vi "Initialize.vi"(8 "error in (no error)":errorcluster, 11 "CCD in":refnum<class "Inclinometer.lvclass">) -> (0 "error out":errorcluster, 3 "CCD out":refnum<class "Inclinometer.lvclass">)   [LabVIEW 2016, in "Hardware.lvlib" / "Inclinometer.lvlib" / "Inclinometer.lvclass"]
uses:
  <userlib>/Common Components/Hardware/Inclinometer/Inclinometer/Inclinometer.lvclass
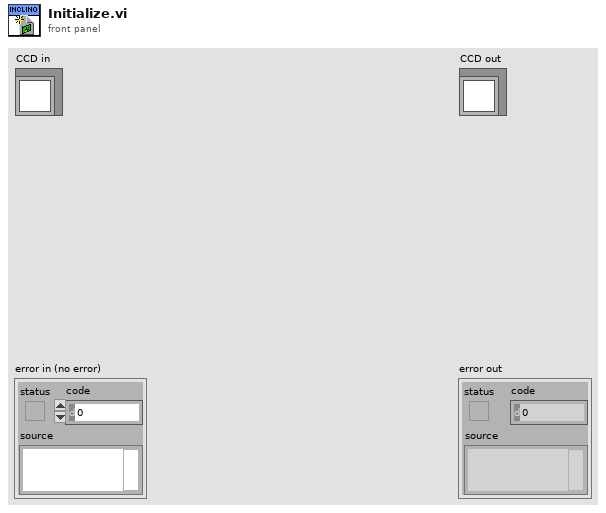
[diagram p1: front panel]
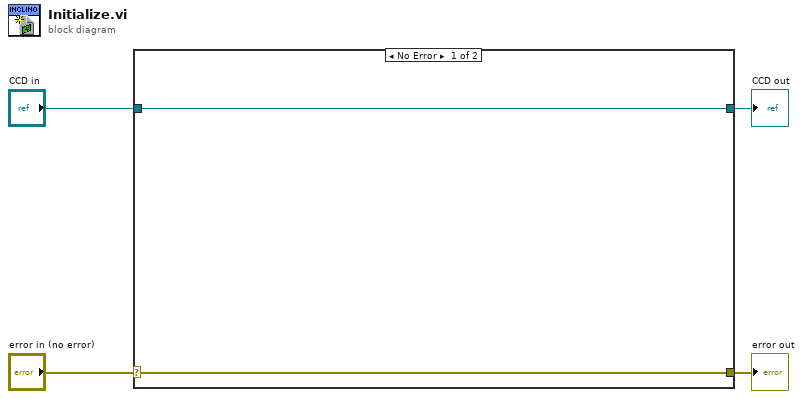
[diagram p0: block diagram]
diagram:
  n1 = case shown="No Error" "error in (no error)" {
    selector: "error in (no error)" -> [w5 w8]
    tunnel: [w5 w8] -> w3
    tunnel: [w6 w7] -> w1
    tunnel: "CCD in" -> [w6 w7]
    frame No Error {
    }
    frame Error {
    }
  }
  "error out" <- w3
  "CCD out" <- w1
